vi "Get Date Time String.vi"() -> (8 "Date Time String":string)   [LabVIEW 2020]
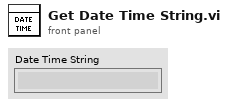
[diagram p1: front panel]
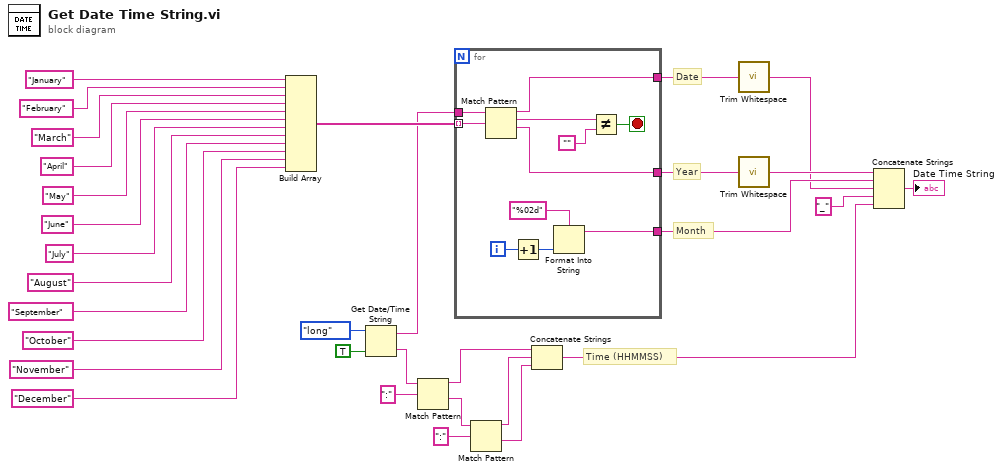
[diagram p0: block diagram]
diagram:
  # "Time (HHMMSS)"
  # "Month"
  # "Year"
  # "Date"
  n1 = Build Array("January" ("regular expression"), "February" ("regular expression"), "March" ("regular expression"), "April" ("regular expression"), "May" ("regular expression"), "June" ("regular expression"), "July" ("regular expression"), "August" ("regular expression"), "September" ("regular expression"), "October" ("regular expression"), "November" ("regular expression"), "December" ("regular expression")) -> (w10:string[])
  n2 = Get Date/Time String(date format (0)=enum16{"short", "long", "abbreviated"}."long", want seconds? (F)=TRUE) -> (date string=w9:string, time string=w24:string)  [unwired: 1 in]
  n3 = Match Pattern(string=w24, regular expression=":") -> (before substring=w26:string, after substring=w29:string)  [unwired: 1 in, 2 out]
  n4 = for {
    tunnel: w10 -> [w41] mode=indexing
    tunnel: w9 -> [w42]
    tunnel: [w34] -> w5
    tunnel: [w33] -> w7
    tunnel: [w32] -> w8
    i -> [w38]
    stop <- w37 stop-if-true
    n5 = Match Pattern(string=w42, regular expression=w41) -> (before substring=w33:string, match substring=w40:string, after substring=w32:string)  [unwired: 1 in, 1 out]
    n6 = Increment(x=w38) -> (x+1=w36:i32)
    n7 = Format Into String(format string="%02d", w36) -> (resulting string=w34:string)  [unwired: 2 in, 1 out]
    n8 = Not Equal?(x=w40, y="") -> (x != y?=w37:bool)
  }
  n9 = Match Pattern(string=w29, regular expression=":") -> (before substring=w30:string, after substring=w31:string)  [unwired: 1 in, 2 out]
  n10 = Concatenate Strings(w26, w30, w31) -> (w2:string)
  n11 = call <vilib>:"Trim Whitespace.vi"("string"=w7) -> ("trimmed string"=w4:string)  [unwired: 1 in]
  n12 = call <vilib>:"Trim Whitespace.vi"("string"=w8) -> ("trimmed string"=w6:string)  [unwired: 1 in]
  n13 = Concatenate Strings(w6, w5, w4, "_", w2) -> (→"Date Time String":string)
